vi "BioFeedback(DAQ+8-channel).vi"(0 "Start Trial":bool, 1 "Moving Average Length (s)":dbl=0.5, 3 "Frames Per Second":dbl=30.0, 4 "Sample rate (Hz)":dbl=1000.0, 5 "End Trial":bool, 9 "Data Directory":path, 11 "End Program":bool, 12 "File Name":string, 13 "VR Data Input File":path=path "C:/Users/Tinggroup/Desktop/VRMuscleActivationVisualizer/StationaryVisualFeedbackVR/assets/BiofeedbackData.txt", 14 "VR Percent Path":path=path "C:/Users/Tinggroup/Desktop/VRMuscleActivationVisualizer/StationaryVisualFeedbackVR/assets/BiofeedbackTargetPercentage.txt") -> (6 "Trial Data":waveform(dbl)(graph), 10 "Moving Avg RMS Graph":dbl(graph), 15 "raw data":dynamicdata(graph))   [LabVIEW 2016]
uses:
  <vilib>/Utility/error.llb/DialogType.ctl
  <vilib>/Analysis/5stat.llb/RMS (DBL).vi
  <vilib>/Waveform/WDTOps.llb/WDT Append Waveforms DBL.vi
  <vilib>/Waveform/WDTFileIO.llb/Export Waveform To Spreadsheet File.vi
  <vilib>/Analysis/NI_AALPro.lvlib
panel:
  out "Moving Avg 1AND2":dbl(slide) scale=0.0..0.01
  out "Moving Avg 3AND4":dbl(slide) scale=0.5..0.7
  out "RMS 3AND4":dbl(graph)
  out "RMS 1AND2":dbl(graph)
  out "RMS 8":dbl(graph)
  out "RMS 7":dbl(graph)
  out "RMS 6":dbl(graph)
  out "RMS 5":dbl(graph)
  out "RMS 4":dbl(graph)
  out "RMS 3":dbl(graph)
  out "RMS 2":dbl(graph)
  out "RMS 1":dbl(graph)
  out "Aggregate8":waveform(dbl)[](array[waveform])
  out "Aggregate7":waveform(dbl)[](array[waveform])
  out "Aggregate6":waveform(dbl)[](array[waveform])
  out "Aggregate5":waveform(dbl)[](array[waveform])
  out "Aggregate4":waveform(dbl)[](array[waveform])
  out "Aggregate3":waveform(dbl)[](array[waveform])
  out "Aggregate2":waveform(dbl)[](array[waveform])
  out "Aggregate1":waveform(dbl)[](array[waveform])
  out "Wfm8":waveform(dbl)
  out "Wfm7":waveform(dbl)
  out "Wfm6":waveform(dbl)
  out "Wfm5":waveform(dbl)
  out "Wfm4":waveform(dbl)
  out "Wfm3":waveform(dbl)
  out "Wfm2":waveform(dbl)
  out "Wfm1":waveform(dbl)
  in  "Extension":string="_EMG.txt"
  in  "Target Percentage":dbl
  out "Trial In Progress":bool
  in  "Trial Number":dbl
  in  "MARK":bool
  out "Moving Avg RMS":dbl(slide) scale=0.0..2.0
  in  "Lower Cut-Off":dbl=20.0
  in  "Upper Cut-Off":dbl=300.0
  out "Bufffer Index":dbl
  out "Frames in Buffer":dbl
  out "Samples per frame":dbl
  out "Reset Data Acquisition\nAnd UI Updating":bool=TRUE
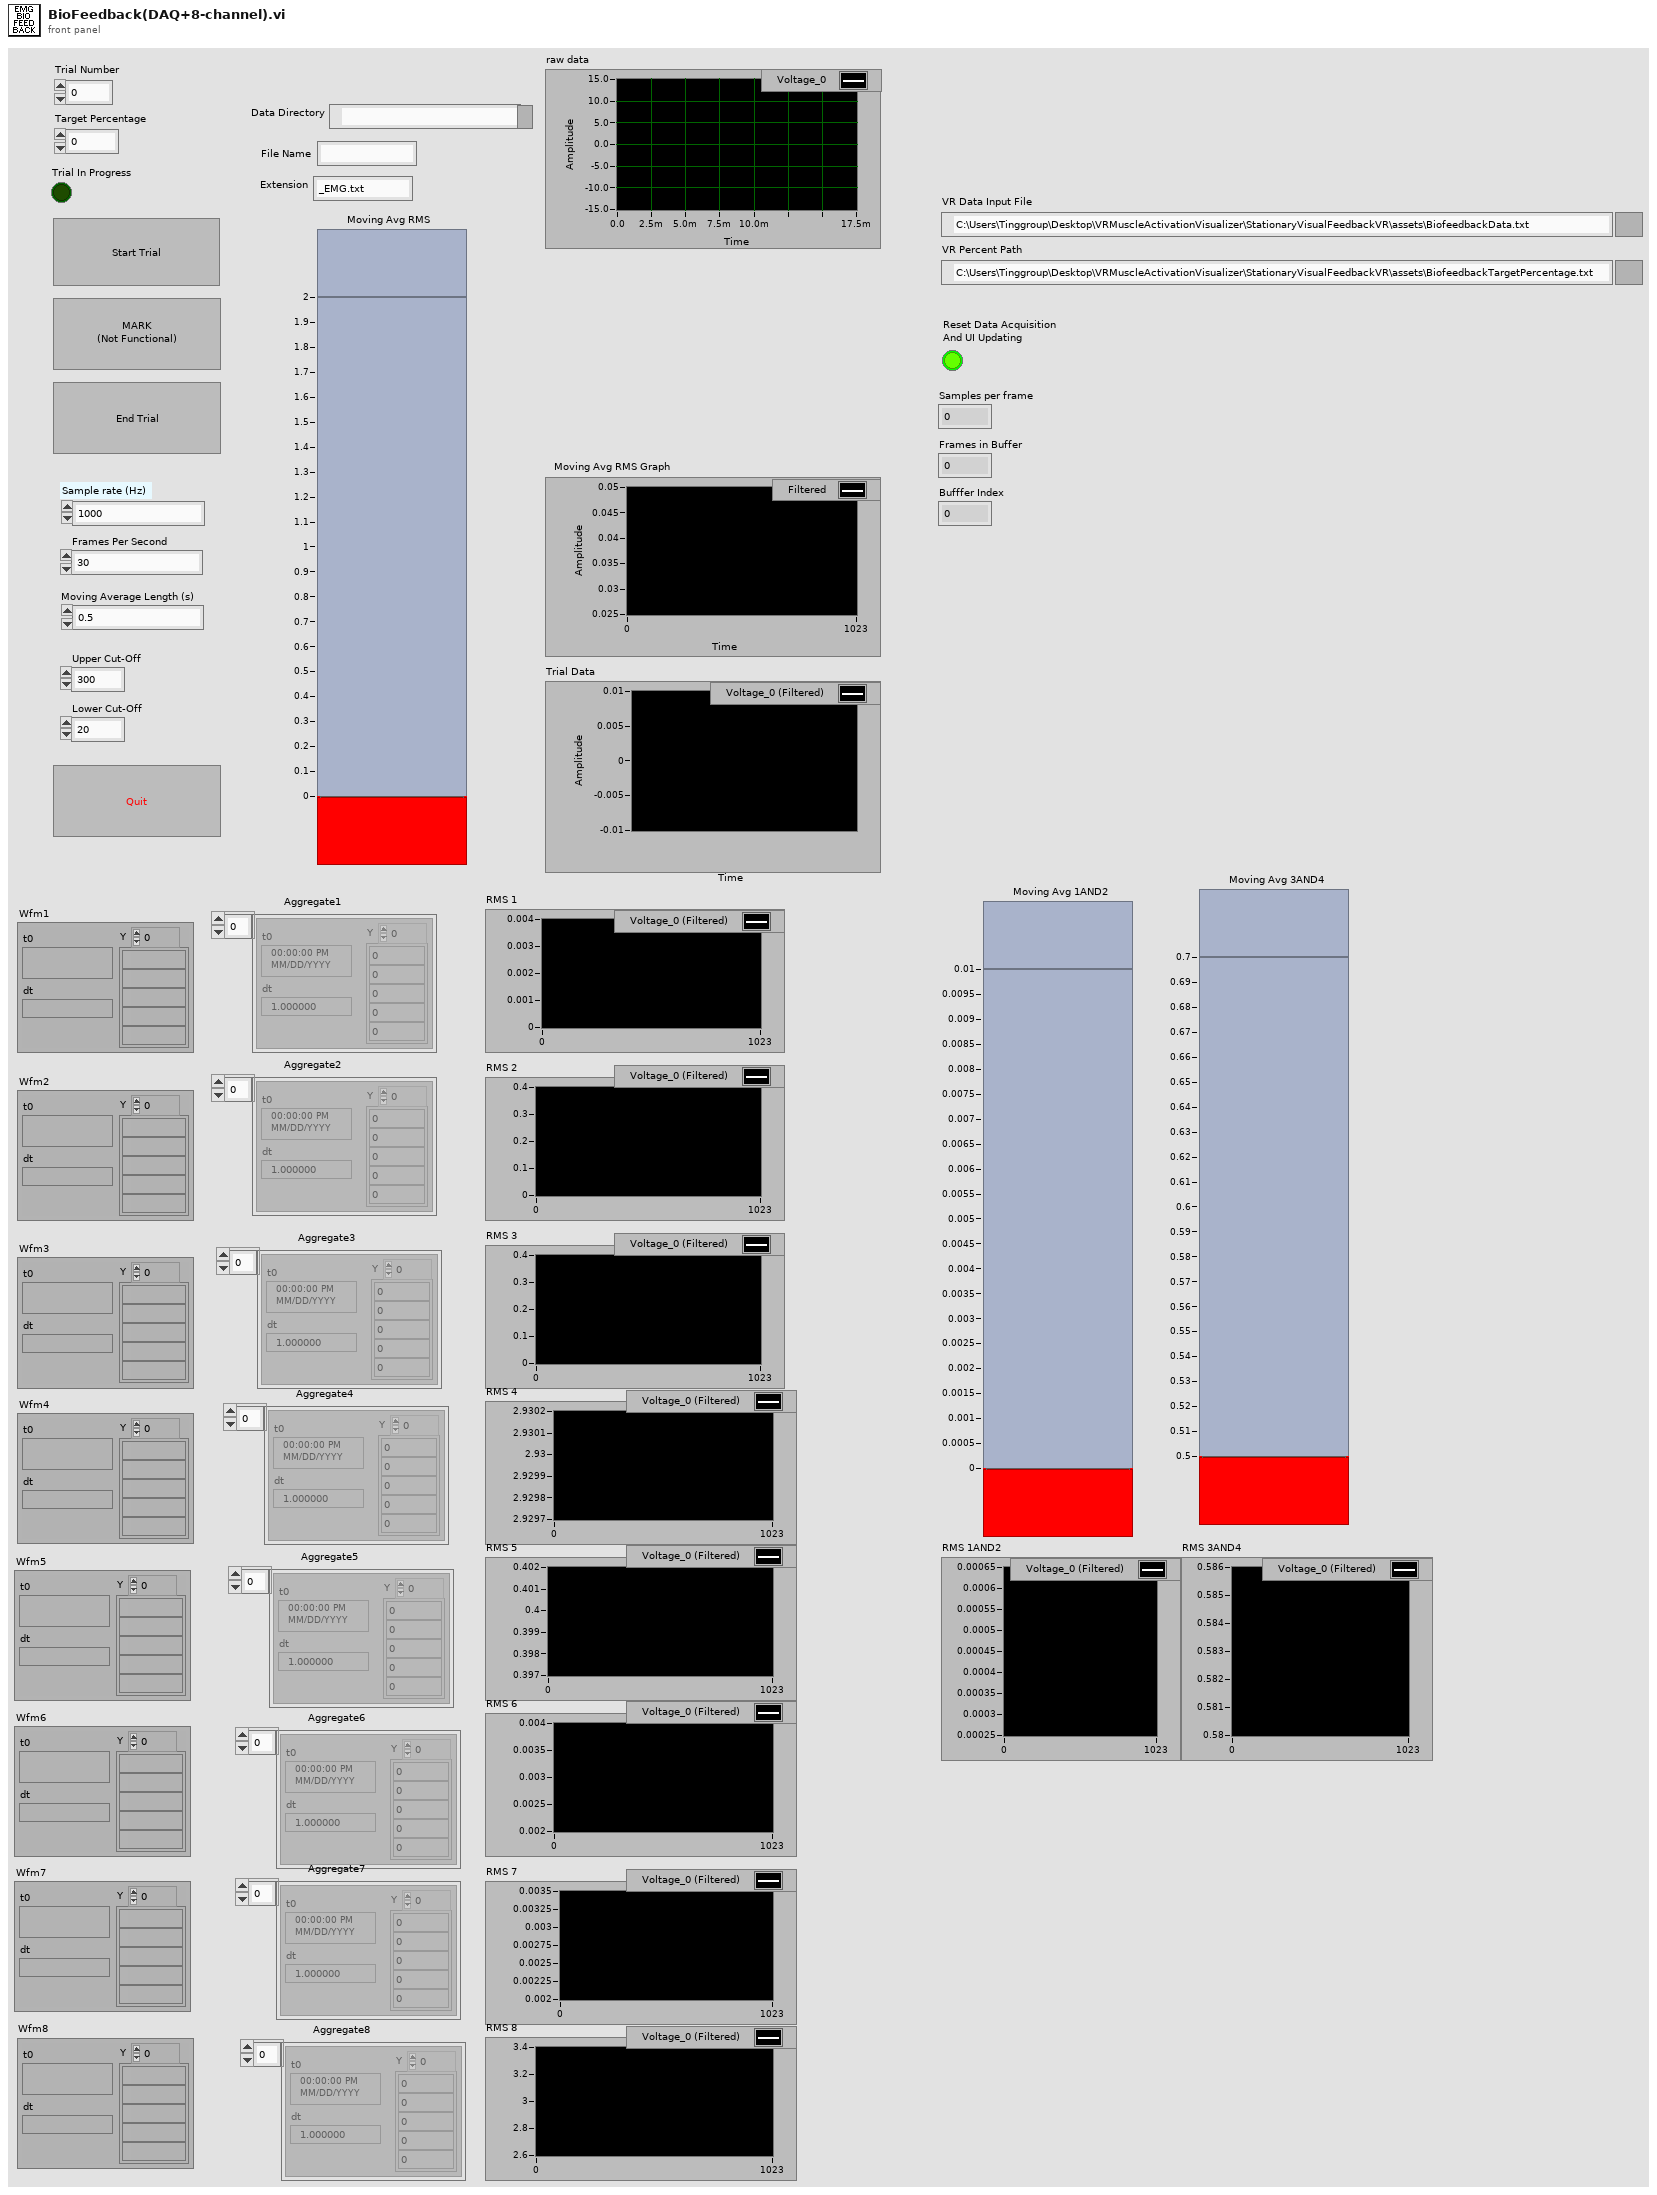
[diagram p1: front panel]
types:
  T1 = typedef "DialogType.ctl" = u16
  T2 = typedef "WaveformArrayControl.ctl" = waveform(dbl)[]
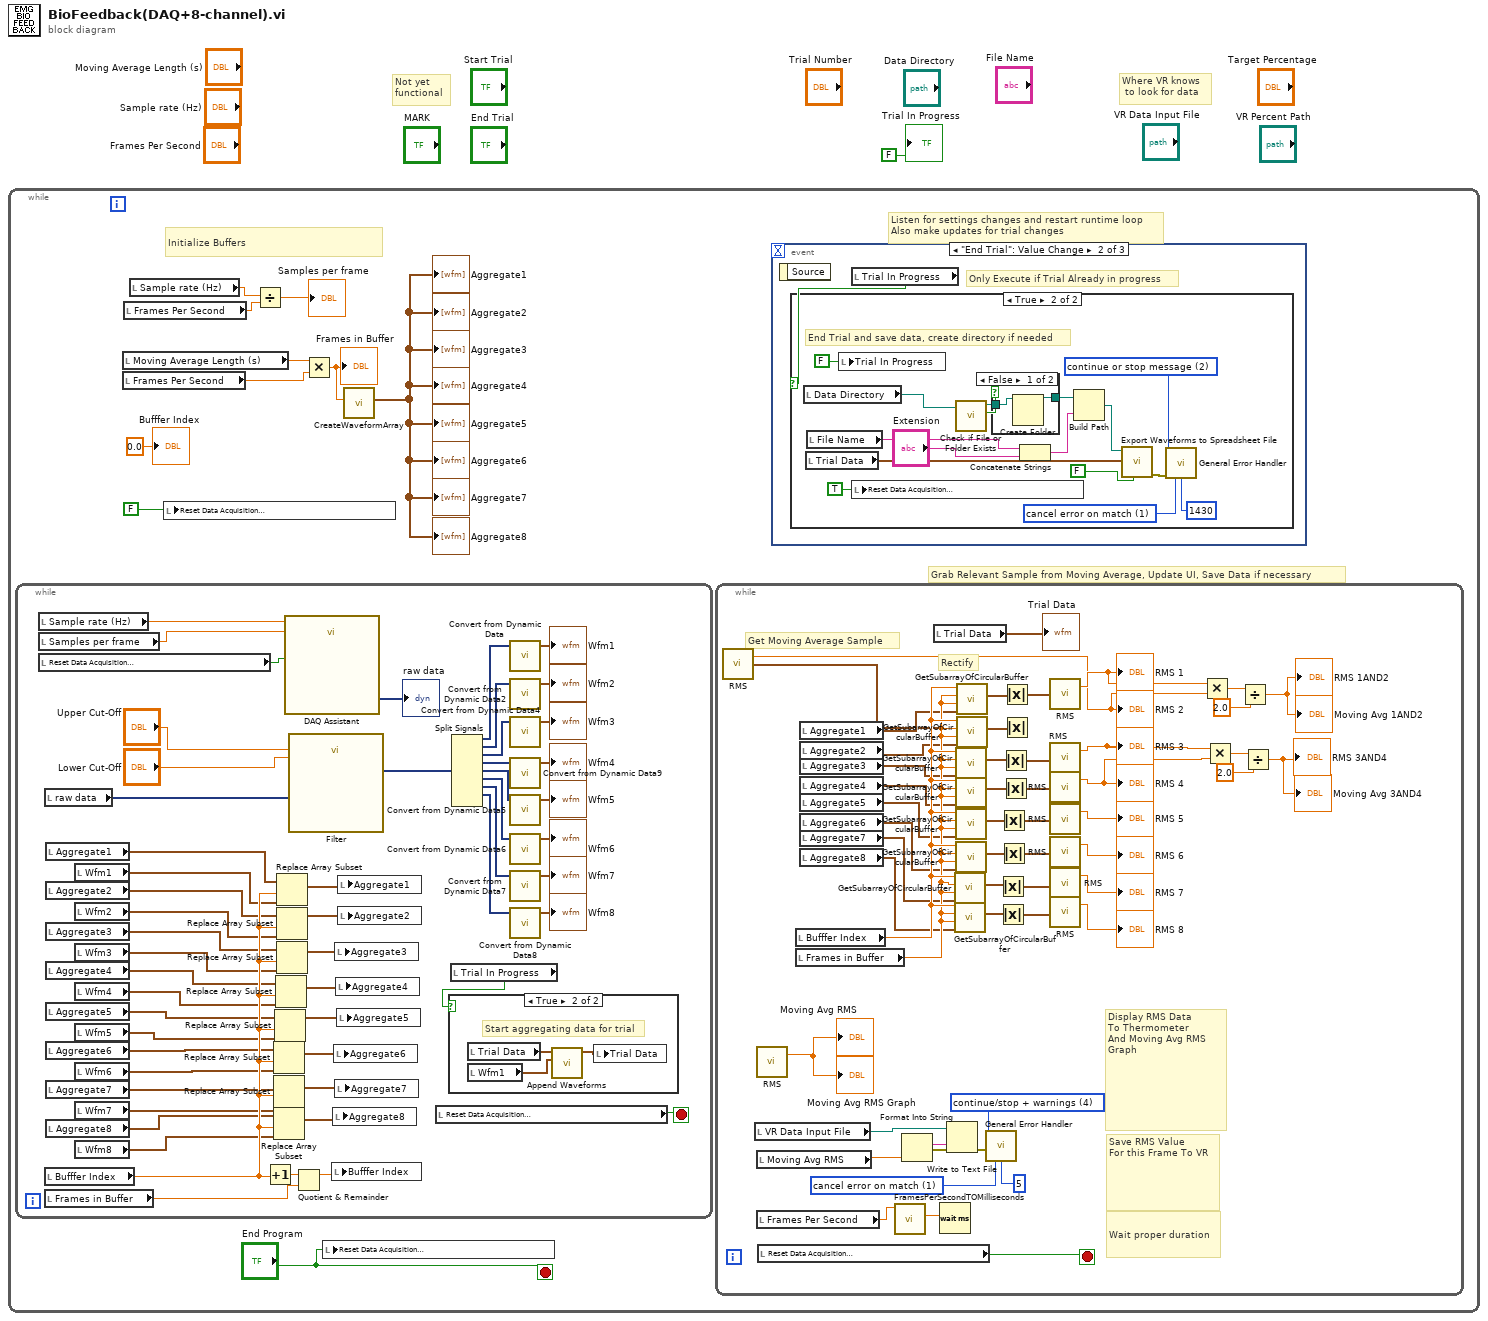
[diagram p0: block diagram]
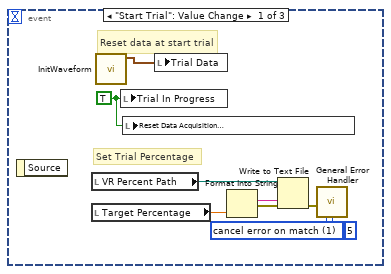
[diagram p2: hidden frame]
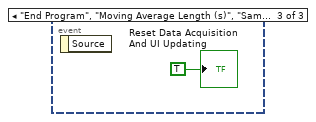
[diagram p5: hidden frame]
diagram:
  # "Not yet \nfunctional"
  # "Where VR knows\n to look for data"
  n1 = while {
    stop <- "End Program" stop-if-true
    # "Grab Relevant Sample from Moving Average, Update UI, Save Data if necessary"
    # "Initialize Buffers"
    # "Listen for settings changes and restart runtime loop\nAlso make updates for trial changes"
    n2 = while {
      stop <- w140 stop-if-true
      n3 = local read "Sample rate (Hz)"() -> (w148:dbl)
      n4 = local read "Samples per frame"() -> (w147:dbl)
      n5 = local read "Reset Data Acquisition\nAnd UI Updating"() -> (w139:bool)
      n6 = local read "raw data"() -> (w145:dynamicdata)
      n7 = local read "Bufffer Index"() -> (w120:dbl)
      n8 = local read "Frames in Buffer"() -> (w142:dbl)
      n9 = local read "Aggregate1"() -> (w119:waveform(dbl)[])
      n10 = local read "Aggregate2"() -> (w117:waveform(dbl)[])
      n11 = local read "Aggregate3"() -> (w115:waveform(dbl)[])
      n12 = local read "Aggregate4"() -> (w113:waveform(dbl)[])
      n13 = local read "Aggregate5"() -> (w111:waveform(dbl)[])
      n14 = local read "Aggregate6"() -> (w109:waveform(dbl)[])
      n15 = local read "Aggregate7"() -> (w107:waveform(dbl)[])
      n16 = local read "Aggregate8"() -> (w105:waveform(dbl)[])
      n17 = local read "Wfm1"() -> (w118:waveform(dbl))
      n18 = local read "Wfm2"() -> (w116:waveform(dbl))
      n19 = local read "Wfm3"() -> (w114:waveform(dbl))
      n20 = local read "Wfm4"() -> (w112:waveform(dbl))
      n21 = local read "Wfm5"() -> (w110:waveform(dbl))
      n22 = local read "Wfm6"() -> (w108:waveform(dbl))
      n23 = local read "Wfm7"() -> (w106:waveform(dbl))
      n24 = local read "Wfm8"() -> (w104:waveform(dbl))
      n25 = Increment(x=w120) -> (x+1=w141:dbl)
      n26 = Replace Array Subset(array=w109, new element=w108, index=w120) -> (w98:waveform(dbl)[])
      n27 = Replace Array Subset(array=w107, new element=w106, index=w120) -> (w97:waveform(dbl)[])
      n28 = Replace Array Subset(array=w105, new element=w104, index=w120) -> (w96:waveform(dbl)[])
      n29 = Replace Array Subset(array=w111, new element=w110, index=w120) -> (w99:waveform(dbl)[])
      n30 = Replace Array Subset(array=w113, new element=w112, index=w120) -> (w100:waveform(dbl)[])
      n31 = Replace Array Subset(array=w119, new element=w118, index=w120) -> (w103:waveform(dbl)[])
      n32 = Replace Array Subset(array=w117, new element=w116, index=w120) -> (w102:waveform(dbl)[])
      n33 = Replace Array Subset(array=w115, new element=w114, index=w120) -> (w101:waveform(dbl)[])
      n34 = call "DAQ Assistant"("rate"=w148, "number of samples"=w147, "stop (T)"=w139) -> ("data"=→"raw data":dynamicdata)  [unwired: 14 in, 2 out]
      n35 = call "Filter"("Lower Cut-Off"="Lower Cut-Off", "Upper Cut-Off"="Upper Cut-Off", "Signal"=w145) -> ("Filtered Signal"=w137:dynamicdata)  [unwired: 7 in, 1 out]
      n36 = Quotient & Remainder(x=w141, y=w142) -> (x-y*floor(x/y)=w143:dbl)  [unwired: 1 out]
      n37 = local write "Bufffer Index"(w143) -> ()
      n38 = local write "Aggregate8"(w96) -> ()
      n39 = local write "Aggregate6"(w98) -> ()
      n40 = local write "Aggregate3"(w101) -> ()
      n41 = local write "Aggregate7"(w97) -> ()
      n42 = local write "Aggregate4"(w100) -> ()
      n43 = local write "Aggregate5"(w99) -> ()
      n44 = local write "Aggregate1"(w103) -> ()
      n45 = local write "Aggregate2"(w102) -> ()
      n46 = local read "Reset Data Acquisition\nAnd UI Updating"() -> (w140:bool)
      n47 = local read "Trial In Progress"() -> (w95:bool)
      n48 = case shown="True" w95 {
        frame False {
        }
        frame True {
          # "Start aggregating data for trial"
          n49 = local read "Trial Data"() -> (w151:waveform(dbl))
          n50 = local read "Wfm1"() -> (w150:waveform(dbl))
          n51 = call-poly <vilib>:"Append Waveforms.vi"("waveform B"=w150, "waveform A"=w151) -> ("waveform out"=w149:waveform(dbl))  [unwired: 8 in, 1 out]
          n52 = local write "Trial Data"(w149) -> ()
        }
      }
      n53 = Split Signals(w137) -> (w136:dynamicdata, w135:dynamicdata, w134:dynamicdata, w133:dynamicdata, w132:dynamicdata, w131:dynamicdata, w130:dynamicdata, w129:dynamicdata)  [unwired: 9 in, 1 out]
      n54 = call "Convert from Dynamic Data"("Dynamic Data Type"=w136) -> ("Waveform"=→"Wfm1":waveform(dbl))  [unwired: 3 in]
      n55 = call "Convert from Dynamic Data2"("Dynamic Data Type"=w135) -> ("Waveform"=→"Wfm2":waveform(dbl))  [unwired: 3 in]
      n56 = call "Convert from Dynamic Data4"("Dynamic Data Type"=w134) -> ("Waveform"=→"Wfm3":waveform(dbl))  [unwired: 3 in]
      n57 = call "Convert from Dynamic Data9"("Dynamic Data Type"=w133) -> ("Waveform"=→"Wfm4":waveform(dbl))  [unwired: 3 in]
      n58 = call "Convert from Dynamic Data5"("Dynamic Data Type"=w132) -> ("Waveform"=→"Wfm5":waveform(dbl))  [unwired: 3 in]
      n59 = call "Convert from Dynamic Data6"("Dynamic Data Type"=w131) -> ("Waveform"=→"Wfm6":waveform(dbl))  [unwired: 3 in]
      n60 = call "Convert from Dynamic Data7"("Dynamic Data Type"=w130) -> ("Waveform"=→"Wfm7":waveform(dbl))  [unwired: 3 in]
      n61 = call "Convert from Dynamic Data8"("Dynamic Data Type"=w129) -> ("Waveform"=→"Wfm8":waveform(dbl))  [unwired: 3 in]
    }
    n62 = local read "Moving Average Length (s)"() -> (w8:dbl)
    n63 = local read "Frames Per Second"() -> (w7:dbl)
    n64 = local read "Frames Per Second"() -> (w10:dbl)
    n65 = local read "Sample rate (Hz)"() -> (w11:dbl)
    n66 = local write "Reset Data Acquisition\nAnd UI Updating"(FALSE) -> ()
    n67 = Divide(x=w11, y=w10) -> (x/y=→"Samples per frame":dbl)
    n68 = Multiply(x=w8, y=w7) -> (x*y=w4:dbl)
    "Frames in Buffer" <- w4
    n69 = local write "Reset Data Acquisition\nAnd UI Updating"("End Program") -> ()
    n70 = call "CreateWaveformArray.vi"("bufferSize"=w4) -> ("initialized array"=→"Aggregate1" →"Aggregate2" →"Aggregate3" →"Aggregate4" →"Aggregate5" →"Aggregate6" →"Aggregate7" →"Aggregate8":waveform(dbl)[])  [unwired: 5 in, 1 out]
    n71 = while {
      stop <- w94 stop-if-true
      w82 = T1 4 items=["no dialog", "OK message", "continue or stop message", "OK message + warnings", "continue/stop + warnings"] ("type of dialog (OK msg:1)")
      w90 = 1 items=["no exception", "cancel error on match", "set error on match"] ("[exception action] (none:0)")
      # "Wait proper duration"
      # "Save RMS Value\nFor this Frame To VR"
      # "Display RMS Data\nTo Thermometer\nAnd Moving Avg RMS\nGraph"
      # "Get Moving Average Sample"
      # "Rectify"
      n72 = local read "VR Data Input File"() -> (w86:path)
      n73 = call-poly <vilib>:"RMS.vi"() -> ("rms value"=→"Moving Avg RMS" →"Moving Avg RMS Graph":dbl)  [unwired: 1 in, 1 out]
      n74 = local read "Moving Avg RMS"() -> (w84:dbl)
      n75 = local read "Frames Per Second"() -> (w92:dbl)
      n76 = local read "Reset Data Acquisition\nAnd UI Updating"() -> (w94:bool)
      n77 = local read "Bufffer Index"() -> (w81:dbl)
      n78 = local read "Frames in Buffer"() -> (w80:dbl)
      n79 = local read "Aggregate1"() -> (w79:waveform(dbl)[])
      n80 = local read "Aggregate2"() -> (w75:waveform(dbl)[])
      n81 = local read "Aggregate3"() -> (w78:waveform(dbl)[])
      n82 = local read "Aggregate4"() -> (w74:waveform(dbl)[])
      n83 = local read "Aggregate5"() -> (w77:waveform(dbl)[])
      n84 = local read "Aggregate6"() -> (w76:waveform(dbl)[])
      n85 = local read "Aggregate7"() -> (w73:waveform(dbl)[])
      n86 = local read "Aggregate8"() -> (w72:waveform(dbl)[])
      n87 = call "FramesPerSecondTOMilliseconds.vi"("Thermometer\nFps"=w92) -> ("x*y"=w91:dbl)  [unwired: 10 in]
      n88 = Format Into String(w84) -> (resulting string=w85:string, error out=w87:errorcluster)  [unwired: 3 in]
      n89 = local read "Trial Data"() -> (→"Trial Data":waveform(dbl))
      n90 = Wait (ms)(milliseconds to wait=w91) -> ()  [unwired: 1 out]
      n91 = Write to Text File(file (use dialog)=w86, text=w85, error in=w87) -> (error out=w88:errorcluster)  [unwired: 1 in, 2 out]
      n92 = call "GetSubarrayOfCircularBuffer.vi"("initialized array"=w73, "buffer size"=w80, "subset size"=w80, "start index"=w81) -> ("initialized array 2"=w65:T2)  [unwired: 7 in]
      n93 = call "GetSubarrayOfCircularBuffer.vi"("initialized array"=w72, "buffer size"=w80, "subset size"=w80, "start index"=w81) -> ("initialized array 2"=w64:T2)  [unwired: 7 in]
      n94 = call "GetSubarrayOfCircularBuffer.vi"("initialized array"=w78, "buffer size"=w80, "subset size"=w80, "start index"=w81) -> ("initialized array 2"=w69:T2)  [unwired: 7 in]
      n95 = call "GetSubarrayOfCircularBuffer.vi"("initialized array"=w74, "buffer size"=w80, "subset size"=w80, "start index"=w81) -> ("initialized array 2"=w68:T2)  [unwired: 7 in]
      n96 = call "GetSubarrayOfCircularBuffer.vi"("initialized array"=w77, "buffer size"=w80, "subset size"=w80, "start index"=w81) -> ("initialized array 2"=w67:T2)  [unwired: 7 in]
      n97 = call "GetSubarrayOfCircularBuffer.vi"("initialized array"=w76, "buffer size"=w80, "subset size"=w80, "start index"=w81) -> ("initialized array 2"=w66:T2)  [unwired: 7 in]
      n98 = call "GetSubarrayOfCircularBuffer.vi"("initialized array"=w79, "buffer size"=w80, "subset size"=w80, "start index"=w81) -> ("initialized array 2"=w71:T2)  [unwired: 7 in]
      n99 = call "GetSubarrayOfCircularBuffer.vi"("initialized array"=w75, "buffer size"=w80, "subset size"=w80, "start index"=w81) -> ("initialized array 2"=w70:T2)  [unwired: 7 in]
      n100 = call <vilib>:"General Error Handler.vi"("type of dialog (OK msg:1)"=w82, "error in (no error)"=w88, "[exception action] (none:0)"=w90, "[exception code]"=5) -> ()  [unwired: 7 in, 5 out]
      n101 = Absolute Value(x=w65) -> (abs(x)=w57:T2)
      n102 = Absolute Value(x=w64) -> (abs(x)=w56:T2)
      n103 = Absolute Value(x=w67) -> (abs(x)=w59:T2)
      n104 = Absolute Value(x=w66) -> (abs(x)=w58:T2)
      n105 = Absolute Value(x=w69) -> (abs(x)=w61:T2)
      n106 = Absolute Value(x=w68) -> (abs(x)=w60:T2)
      n107 = Absolute Value(x=w71) -> (abs(x)=w63:T2)
      n108 = Absolute Value(x=w70) -> (abs(x)=w62:T2)
      n109 = call-poly <vilib>:"RMS.vi"("X"=w62) -> ("rms value"=w50:dbl)  [unwired: 1 out]
      "RMS 2" <- w50
      n110 = call-poly <vilib>:"RMS.vi"("X"=w63) -> ("rms value"=w51:dbl)  [unwired: 1 out]
      "RMS 1" <- w51
      n111 = call-poly <vilib>:"RMS.vi"("X"=w61) -> ("rms value"=w45:dbl)  [unwired: 1 out]
      "RMS 3" <- w45
      n112 = call-poly <vilib>:"RMS.vi"("X"=w60) -> ("rms value"=w44:dbl)  [unwired: 1 out]
      "RMS 4" <- w44
      n113 = call-poly <vilib>:"RMS.vi"("X"=w59) -> ("rms value"=→"RMS 5":dbl)  [unwired: 1 out]
      n114 = call-poly <vilib>:"RMS.vi"("X"=w58) -> ("rms value"=→"RMS 6":dbl)  [unwired: 1 out]
      n115 = call-poly <vilib>:"RMS.vi"("X"=w57) -> ("rms value"=→"RMS 7":dbl)  [unwired: 1 out]
      n116 = call-poly <vilib>:"RMS.vi"("X"=w56) -> ("rms value"=→"RMS 8":dbl)  [unwired: 1 out]
      n117 = Multiply(x=w51, y=w50) -> (x*y=w49:dbl)
      n118 = Multiply(x=w45, y=w44) -> (x*y=w47:dbl)
      n119 = Divide(x=w49, y=2.0) -> (x/y=→"RMS 1AND2" →"Moving Avg 1AND2":dbl)
      n120 = Divide(x=w47, y=2.0) -> (x/y=→"RMS 3AND4" →"Moving Avg 3AND4":dbl)
    }
    n121 = event shown="[1] \"End Trial\": Value Change" {
      selector: _ -> [_ _ _]
      dyn-events: _ -> [_ _ _]
      timeout: _ -> [_ _ _]
      event "Start Trial": Value Change {
        w18 = 1 items=["no exception", "cancel error on match", "set error on match"] ("[exception action] (none:0)")
        w19 = TRUE ("Trial In Progress")
        # "Set Trial Percentage"
        # "Reset data at start trial"
        n122 = event-data() -> ()  [unwired: 1 in, 1 out]
        n123 = local read "VR Percent Path"() -> (w13:path)
        n124 = local read "Target Percentage"() -> (w12:dbl)
        n125 = call "InitWaveform.vi"() -> ("output waveform"=w20:waveform(dbl))  [unwired: 11 in]
        n126 = local write "Trial In Progress"(w19) -> ()
        n127 = local write "Reset Data Acquisition\nAnd UI Updating"(w19) -> ()
        n128 = local write "Trial Data"(w20) -> ()
        n129 = Format Into String(w12) -> (resulting string=w14:string, error out=w15:errorcluster)  [unwired: 3 in]
        n130 = Write to Text File(file (use dialog)=w13, text=w14, error in=w15) -> (error out=w16:errorcluster)  [unwired: 1 in, 2 out]
        n131 = call <vilib>:"General Error Handler.vi"("error in (no error)"=w16, "[exception action] (none:0)"=w18, "[exception code]"=5) -> ()  [unwired: 8 in, 5 out]
      }
      event "End Trial": Value Change {
        # "Only Execute if Trial Already in progress"
        n132 = event-data() -> ()  [unwired: 1 in, 1 out]
        n133 = local read "Trial In Progress"() -> (w21:bool)
        n134 = case shown="True" w21 {
          frame False {
          }
          frame True {
            w30 = T1 2 items=["no dialog", "OK message", "continue or stop message", "OK message + warnings", "continue/stop + warnings"] ("type of dialog (OK msg:1)")
            w31 = 1 items=["no exception", "cancel error on match", "set error on match"] ("[exception action] (none:0)")
            # "End Trial and save data, create directory if needed"
            n135 = local read "Data Directory"() -> (w33:path)
            n136 = local read "Trial Data"() -> (w25:waveform(dbl))
            n137 = local read "File Name"() -> (w28:string)
            n138 = local write "Trial In Progress"(FALSE ("Trial In Progress")) -> ()
            n139 = local write "Reset Data Acquisition\nAnd UI Updating"(TRUE ("Reset Data Acquisition\nAnd UI Updating")) -> ()
            n140 = call <vilib>:"Check if File or Folder Exists.vi"("path"=w33) -> ("file or folder exists?"=w35:bool, "dup path"=w34:path)  [unwired: 8 in, 1 out]
            n141 = case shown="False" w35 {
              tunnel: [w38 w40] -> w26
              tunnel: w34 -> [w39 w40]
              frame False {
                n142 = Create Folder(path (use dialog)=w39) -> (created path=w38:path)  [unwired: 2 in, 2 out]
              }
              frame True {
              }
            }
            n143 = Concatenate Strings(w28, "Extension") -> (w27:string)
            n144 = Build Path(base path=w26, name or relative path=w27) -> (appended path=w24:path)
            n145 = call-poly <vilib>:"Export Waveforms to Spreadsheet File.vi"("append to file? (new file:F)"=FALSE, "waveform"=w25, "file path (dialog if empty)"=w24) -> ("error out"=w23:errorcluster)  [unwired: 7 in, 1 out]
            n146 = call <vilib>:"General Error Handler.vi"("type of dialog (OK msg:1)"=w30, "error in (no error)"=w23, "[exception action] (none:0)"=w31, "[exception code]"=1430) -> ()  [unwired: 7 in, 5 out]
          }
        }
      }
      event "End Program", "Moving Average Length (s)", "Sample rate (Hz)", "Frames Per Second": Value Change {
        n147 = event-data() -> ()  [unwired: 1 in, 1 out]
        "Reset Data Acquisition\nAnd UI Updating" <- TRUE
      }
    }
    "Bufffer Index" <- 0.0 ("Bufffer Index")
  }
  "Trial In Progress" <- FALSE ("Trial In Progress")
